vi "log analysis_gps.vi"() -> ()   [LabVIEW 2018] (continued)
normal 2 28.000000 0 0\trobot status\t244.692862\t98.039644\t8.450300\t-0.803805\t-0.502559\t154.815387\t0.298000\t0.012000\n\t\n15:36:08.1\tlog_raw\tgps_raw\t#INSPVAXA,USB3,0,46.5,FINESTEERING,2107,282986.150,02008000,471d,15824;INS_ALIGNMENT_COMPLETE,INS_RTKFIXED,37.37101422818,126.72359615090,8.4473,22.3000,0.1631,-0.2437,-0.0170,-1.039180574,-0.597901795,295.266800009,0.4472,0.2951,0.5600,0.1141,0.0926,0.0776,0.0978,0.1028,4.9255,0f000001,0*b918d4c4\n\tsystem status\tnormal 2 28.000000 0 0\trobot status\t244.568915\t98.110325\t8.447300\t-1.039181\t-0.597902\t154.733200\t0.361000\t-0.105000\n\t\n15:36:08.6\tlog_raw\tgps_raw\t\tsystem status\tnormal 2 27.900000 0 0\trobot status\t244.444418\t98.179771\t8.446900\t-1.452290\t-0.735471\t154.720591\t0.349000\t-0.074000\n\t\n15:36:09.1\tlog_raw\tgps_raw\t\tsystem status\tnormal 2 27.900000 0 0\trobot status\t244.323302\t98.251356\t8.447400\t-1.387904\t-0.757629\t154.772005\t0.295000\t0.004000\n\t\n15:36:09.6\tlog_raw\tgps_raw\t\tsystem status\tnormal 2 27.900000 0 0\trobot status\t244.200377\t98.324148\t8.445900\t-1.199779\t-0.776977\t154.794421\t0.351000\t-0.085000\n\t\n15:36:10.1\tlog_raw\tgps_raw\t#INSPVAXA,USB3,0,51.5,FINESTEERING,2107,282988.150,02000000,471d,15824;INS_ALIGNMENT_COMPLETE,INS_RTKFIXED,37.37101680407,126.72359058877,8.4432,22.3000,0.1712,-0.2477,-0.0072,-1.132987341,-0.795555306,295.241601401,0.4472,0.2951,0.5599,0.1141,0.0926,0.0776,0.0978,0.1028,4.9272,0f000001,0*1b3b971d\n\tsystem status\tnormal 2 28.000000 0 0\trobot status\t244.076230\t98.396223\t8.443200\t-1.132987\t-0.795555\t154.758399\t0.259000\t0.061000\n\t\n15:36:10.6\tlog_raw\tgps_raw\t#INSPVAXA,USB3,0,51.5,FINESTEERING,2107,282988.650,02000000,471d,15824;INS_ALIGNMENT_COMPLETE,INS_RTKFIXED,37.37101744623,126.72358920504,8.4402,22.3000,0.1681,-0.2455,-0.0077,-0.918184944,-0.964879494,295.259837239,0.4472,0.2951,0.5599,0.1141,0.0926,0.0776,0.0978,0.1028,4.9272,0f000001,0*72c9ff23\n\tsystem status\tnormal 2 27.900000 0 0\trobot status\t243.953662\t98.467497\t8.440200\t-0.918185\t-0.964879\t154.740163\t0.282000\t0.015000\n\t\n15:36:11.1\tlog_raw\tgps_raw\t#INSPVAXA,USB3,0,52.0,FINESTEERING,2107,282989.150,02000000,471d,15824;INS_ALIGNMENT_COMPLETE,INS_RTKFIXED,37.37101810010,126.72358780342,8.4378,22.3000,0.1635,-0.2346,-0.0127,-0.821579606,-1.181208357,295.261813725,0.4470,0.2950,0.5598,0.1141,0.0925,0.0776,0.0977,0.1028,4.9279,0f000001,0*084187d8\n\tsystem status\tnormal 2 27.900000 0 0\trobot status\t243.829509\t98.540070\t8.437800\t-0.821580\t-1.181208\t154.738186\t0.346000\t-0.094000\n\t\n15:36:11.6\tlog_raw\tgps_raw\t#INSPVAXA,USB3,0,52.0,FINESTEERING,2107,282989.650,02000000,471d,15824;INS_ALIGNMENT_COMPLETE,INS_RTKFIXED,37.37101876823,126.72358639475,8.4359,22.3000,0.1596,-0.2371,-0.0062,-0.715677130,-1.181942284,295.239523711,0.4470,0.2950,0.5598,0.1141,0.0925,0.0776,0.0977,0.1028,4.9279,0f000001,0*db6d0e7d\n\tsystem status\tnormal 2 28.000000 0 0\trobot status\t243.704731\t98.614226\t8.435900\t-0.715677\t-1.181942\t154.760476\t0.253000\t0.047000\n\t\n15:36:12.1\tlog_raw\tgps_raw\t#INSPVAXA,USB3,0,50.0,FINESTEERING,2107,282990.150,02000000,471d,15824;INS_ALIGNMENT_COMPLETE,INS_RTKFIXED,37.37101943584,126.72358497714,8.4335,22.3000,0.1613,-0.2440,-0.0113,-0.746627018,-1.102743180,295.224075586,0.4466,0.2950,0.5597,0.1141,0.0925,0.0776,0.0977,0.1028,4.9289,0f000001,0*6b0a1647\n\tsystem status\tnormal 2 28.000000 0 0\trobot status\t243.579161\t98.688324\t8.433500\t-0.746627\t-1.102743\t154.775924\t0.282000\t0.033000\n\t\n15:36:12.6\tlog_raw\tgps_raw\t#INSPVAXA,USB3,0,50.0,FINESTEERING,2107,282990.650,02000000,471d,15824;INS_ALIGNMENT_COMPLETE,INS_RTKFIXED,37.37102009853,126.72358357998,8.4311,22.3000,0.1630,-0.2513,-0.0092,-0.640841059,-0.917447835,295.078324917,0.4466,0.2950,0.5597,0.1141,0.0925,0.0776,0.0977,0.1028,4.9289,0f000001,0*b9d8443c\n\tsystem status\tnormal 2 28.000000 0 0\trobot status\t243.455403\t98.761876\t8.431100\t-0.640841\t-0.917448\t154.921675\t0.378000\t-0.109000\n\t\n15:36:13.1\tlog_raw\tgps_raw\t#INSPVAXA,USB3,0,51.0,FINESTEERING,2107,282991.150,02000000,471d,15824;INS_ALIGNMENT_COMPLETE,INS_RTKFIXED,37.37102077697,126.72358217095,8.4272,22.3000,0.1498,-0.2404,-0.0111,-0.329986353,-0.737306515,294.974204977,0.4460,0.2950,0.5595,0.1141,0.0925,0.0776,0.0977,0.1028,4.9303,0f000001,0*44f52417\n\tsystem status\tnormal 2 27.900000 0 0\trobot status\t243.330594\t98.837176\t8.427200\t-0.329986\t-0.737307\t155.025795\t0.275000\t0.036000\n\t\n15:36:13.6\tlog_raw\tgps_raw\t\tsystem status\tnormal 2 27.900000 0 0\trobot status\t243.204049\t98.910416\t8.424600\t-0.403055\t-0.840461\t155.109599\t0.256000\t0.075000\n\t\n15:36:14.1\tlog_raw\tgps_raw\t#INSPVAXA,USB3,0,52.0,FINESTEERING,2107,282992.150,02000000,471d,15824;INS_ALIGNMENT_COMPLETE,INS_RTKFIXED,37.37102208780,126.72357933244,8.4219,22.3000,0.1505,-0.2512,-0.0006,-0.471923349,-0.884947239,294.718584068,0.4460,0.2949,0.5594,0.1141,0.0926,0.0776,0.0977,0.1028,4.9317,0f000001,0*525866c6\n\tsystem status\tnormal 2 27.900000 0 0\trobot status\t243.079163\t98.982665\t8.421900\t-0.471923\t-0.884947\t155.281416\t0.245000\t0.082000\n\t\n15:36:14.6\tlog_raw\tgps_raw\t\tsystem status\tnormal 2 27.900000 0 0\trobot status\t242.954926\t99.054298\t8.420600\t-0.447132\t-0.873245\t155.408066\t0.286000\t0.033000\n\t\n15:36:15.1\tlog_raw\tgps_raw\t\tsystem status\tnormal 2 27.900000 0 0\trobot status\t242.830833\t99.126924\t8.419200\t-0.327815\t-0.760203\t155.517928\t0.356000\t-0.079000\n\t\n15:36:15.6\tlog_raw\tgps_raw\t\tsystem status\tnormal 2 27.900000 0 0\trobot status\t242.705129\t99.198573\t8.417700\t-0.367400\t-0.721993\t155.690211\t0.279000\t0.039000\n\t\n15:36:16.1\tlog_raw\tgps_raw\t\tsystem status\tnormal 2 27.900000 0 0\trobot status\t242.579117\t99.269179\t8.416000\t-0.582357\t-0.735126\t155.797376\t0.243000\t0.086000\n\t\n15:36:16.6\tlog_raw\tgps_raw\t\tsystem status\tnormal 2 27.900000 0 0\trobot status\t242.453519\t99.339670\t8.415000\t-0.617090\t-0.662184\t155.942723\t0.354000\t-0.074000\n\t\n15:36:17.1\tlog_raw\tgps_raw\t\tsystem status\tnormal 2 27.900000 0 0\trobot status\t242.325366\t99.411603\t8.413900\t-0.531047\t-0.781812\t156.112555\t0.222000\t0.108000\n\t\n15:36:17.6\tlog_raw\tgps_raw\t\tsystem status\tnormal 2 27.900000 0 0\trobot status\t242.197882\t99.480396\t8.412000\t-0.574216\t-0.924224\t156.274601\t0.281000\t0.029000\n\t\n15:36:18.1\tlog_raw\tgps_raw\t\tsystem status\tnormal 2 27.900000 0 0\trobot status\t242.070413\t99.549648\t8.409200\t-0.560898\t-1.025999\t156.424077\t0.327000\t-0.033000\n\t\n15:36:18.6\tlog_raw\tgps_raw\t\tsystem status\tnormal 2 27.900000 0 0\trobot status\t241.941493\t99.617825\t8.405800\t-0.542524\t-1.180480\t156.491955\t0.254000\t0.064000\n\t\n15:36:19.1\tlog_raw\tgps_raw\t\tsystem status\tnormal 2 27.900000 0 0\trobot status\t241.811834\t99.686587\t8.402800\t-0.566001\t-1.561653\t156.587783\t0.260000\t0.056000\n\t\n15:36:19.6\tlog_raw\tgps_raw\t\tsystem status\tnormal 2 27.900000 0 0\trobot status\t241.684911\t99.755728\t8.400600\t-0.615139\t-1.607167\t156.703459\t0.290000\t0.026000\n\t\n15:36:20.1\tlog_raw\tgps_raw\t\tsystem status\tnormal 2 27.900000 0 0\trobot status\t241.559726\t99.825209\t8.399300\t-0.552219\t-1.574627\t156.768165\t0.262000\t0.066000\n\t\n15:36:20.6\tlog_raw\tgps_raw\t\tsystem status\tnormal 2 27.900000 0 0\trobot status\t241.433525\t99.894376\t8.397900\t-0.537757\t-1.498689\t156.817308\t0.339000\t-0.045000\n\t\n15:36:21.1\tlog_raw\tgps_raw\t\tsystem status\tnormal 2 27.900000 0 0\trobot status\t241.309976\t99.962850\t8.395200\t-0.464581\t-1.180262\t156.857945\t0.334000\t-0.044000\n\t\n15:36:21.6\tlog_raw\tgps_raw\t\tsystem status\tnormal 2 27.900000 0 0\trobot status\t241.187325\t100.030799\t8.392900\t-0.376983\t-1.123165\t156.922194\t0.223000\t0.121000\n\t\n15:36:22.1\tlog_raw\tgps_raw\t#INSPVAXA,USB3,0,42.5,FINESTEERING,2107,283000.150,02008000,471d,15824;INS_ALIGNMENT_COMPLETE,INS_RTKFIXED,37.37103215127,126.72355655993,8.3901,22.3000,0.1524,-0.2449,-0.0003,-0.362652962,-1.080137119,293.057786334,0.4445,0.2951,0.5592,0.1140,0.0926,0.0776,0.0977,0.1028,4.9425,0f000001,0*4235a1eb\n\tsystem status\tnormal 2 28.000000 0 0\trobot status\t241.062012\t100.099614\t8.390100\t-0.362653\t-1.080137\t156.942214\t0.357000\t-0.096000\n\t\n15:36:22.6\tlog_raw\tgps_raw\t\tsystem status\tnormal 2 28.000000 0 0\trobot status\t240.934705\t100.169062\t8.388500\t-0.314213\t-1.316526\t156.995133\t0.237000\t0.069000\n\t\n15:36:23.1\tlog_raw\tgps_raw\t\tsystem status\tnormal 2 28.000000 0 0\trobot status\t240.809010\t100.237494\t8.386700\t-0.267509\t-1.341608\t157.070363\t0.307000\t0.007000\n\t\n15:36:23.6\tlog_raw\tgps_raw\t\tsystem status\tnormal 2 27.900000 0 0\trobot status\t240.686600\t100.302527\t8.386000\t-0.209028\t-1.240600\t157.178946\t0.374000\t-0.108000\n\t\n15:36:24.1\tlog_raw\tgps_raw\t\tsystem status\tnormal 2 27.900000 0 0\trobot status\t240.561796\t100.368931\t8.383800\t-0.114387\t-1.159675\t157.312989\t0.298000\t-0.019000\n\t\n15:36:24.6\tlog_raw\tgps_raw\t\tsystem status\tnormal 2 27.900000 0 0\trobot status\t240.435903\t100.435393\t8.381400\t-0.172130\t-1.043551\t157.446511\t0.220000\t0.117000\n\t\n15:36:25.1\tlog_raw\tgps_raw\t\tsystem status\tnormal 2 27.900000 0 0\trobot status\t240.309740\t100.501734\t8.378200\t-0.129443\t-1.017241\t157.594683\t0.348000\t-0.088000\n\t\n15:36:25.6\tlog_raw\tgps_raw\t#INSPVAXA,USB3,0,49.0,FINESTEERING,2107,283003.650,02008000,471d,15824;INS_ALIGNMENT_COMPLETE,INS_RTKFIXED,37.37103636428,126.72354662832,8.3755,22.3000,0.1350,-0.2615,-0.0053,-0.069883534,-0.948015743,292.302597203,0.4446,0.2951,0.5590,0.1140,0.0925,0.0776,0.0978,0.1028,4.9465,0f000001,0*59130eb8\n\tsystem status\tnormal 2 27.900000 0 0\trobot status\t240.182286\t100.567218\t8.375500\t-0.069884\t-0.948016\t157.697403\t0.347000\t-0.082000\n\t\n15:36:26.1\tlog_raw\tgps_raw\t\tsystem status\tnormal 2 27.900000 0 0\trobot status\t240.051657\t100.633146\t8.372800\t-0.173374\t-1.126467\t157.829281\t0.280000\t0.015000\n\t\n15:36:26.7\tlog_raw\tgps_raw\t\tsystem status\tnormal 2 27.900000 0 0\trobot status\t239.922071\t100.698890\t8.370700\t-0.264071\t-1.188422\t158.025138\t0.283000\t0.034000\n\t\n15:36:27.2\tlog_raw\tgps_raw\t\tsystem status\tnormal 2 27.900000 0 0\trobot status\t239.792839\t100.765236\t8.368100\t-0.305352\t-1.271586\t158.094882\t0.339000\t-0.062000\n\t\n15:36:27.6\tlog_raw\tgps_raw\t\tsystem status\tnormal 2 27.900000 0 0\trobot status\t239.663623\t100.830918\t8.366100\t-0.343211\t-1.324235\t158.195980\t0.450000\t-0.229000\n\t\n15:36:28.2\tlog_raw\tgps_raw\t\tsystem status\tnormal 2 27.900000 0 0\trobot status\t239.534352\t100.896705\t8.364200\t-0.314060\t-1.319994\t158.324136\t0.257000\t0.072000\n\t\n15:36:28.7\tlog_raw\tgps_raw\t\tsystem status\tnormal 2 27.900000 0 0\trobot status\t239.406547\t100.960925\t8.362500\t-0.258928\t-1.174312\t158.404351\t0.381000\t-0.103000\n\t\n15:36:29.1\tlog_raw\tgps_raw\t\tsystem status\tnormal 2 27.900000 0 0\trobot status\t239.277688\t101.025267\t8.359900\t-0.293969\t-1.010654\t158.496365\t0.346000\t-0.059000\n\t\n15:36:29.6\tlog_raw\tgps_raw\t\tsystem status\tnormal 2 27.900000 0 0\trobot status\t239.148045\t101.088847\t8.357100\t-0.431958\t-0.959264\t158.582891\t0.287000\t0.019000\n\t\n15:36:30.2\tlog_raw\tgps_raw\t\tsystem status\tnormal 2 27.900000 0 0\trobot status\t239.019804\t101.152841\t8.355200\t-0.465469\t-0.805617\t158.766817\t0.372000\t-0.098000\n\t\n15:36:30.6\tlog_raw\tgps_raw\t\tsystem status\tnormal 2 27.900000 0 0\trobot status\t238.892777\t101.217417\t8.354000\t-0.368318\t-0.774393\t158.922796\t0.341000\t-0.059000\n\t\n15:36:31.1\tlog_raw\tgps_raw\t\tsystem status\tnormal 2 27.900000 0 0\trobot status\t238.763580\t101.282027\t8.352100\t-0.373752\t-0.757788\t159.085038\t0.222000\t0.122000\n\t\n15:36:31.7\tlog_raw\tgps_raw\t\tsystem status\tnormal 2 27.900000 0 0\trobot status\t238.634583\t101.344929\t8.350300\t-0.519696\t-0.590256\t159.213603\t0.342000\t-0.067000\n\t\n15:36:32.2\tlog_raw\tgps_raw\t\tsystem status\tnormal 2 27.900000 0 0\trobot status\t238.504480\t101.407745\t8.349200\t-0.610956\t-0.693965\t159.324003\t0.224000\t0.115000\n\t\n15:36:32.6\tlog_raw\tgps_raw\t\tsystem status\tnormal 2 27.900000 0 0\trobot status\t238.374891\t101.469502\t8.348000\t-0.622591\t-0.731069\t159.487231\t0.209000\t0.143000\n\t\n15:36:33.1\tlog_raw\tgps_raw\t\tsystem status\tnormal 2 27.900000 0 0\trobot status\t238.244641\t101.530850\t8.346700\t-0.723407\t-0.771971\t159.667053\t0.366000\t-0.093000\n\t\n15:36:33.7\tlog_raw\tgps_raw\t\tsystem status\tnormal 2 27.900000 0 0\trobot status\t238.115486\t101.591392\t8.347000\t-0.788066\t-0.747634\t159.858332\t0.281000\t0.037000\n\t\n15:36:34.1\tlog_raw\tgps_raw\t\tsystem status\tnormal 2 27.900000 0 0\trobot status\t237.986285\t101.650207\t8.346900\t-0.994357\t-0.650902\t159.990881\t0.215000\t0.129000\n\t\n15:36:34.6\tlog_raw\tgps_raw\t\tsystem status\tnormal 2 27.900000 0 0\trobot status\t237.858246\t101.709402\t8.345300\t-1.038620\t-0.473997\t160.049241\t0.248000\t0.082000\n\t\n15:36:35.2\tlog_raw\tgps_raw\t\tsystem status\tnormal 2 27.900000 0 0\trobot status\t237.728450\t101.768656\t8.343900\t-1.062118\t-0.508142\t160.161998\t0.278000\t0.032000\n\t\n15:36:35.7\tlog_raw\tgps_raw\t\tsystem status\tnormal 2 28.000000 0 0\trobot status\t237.599188\t101.827012\t8.344700\t-1.031691\t-0.580801\t160.225175\t0.210000\t0.139000\n\t\n15:36:36.2\tlog_raw\tgps_raw\t\tsystem status\tnormal 2 27.900000 0 0\trobot status\t237.468929\t101.885123\t8.345300\t-1.104431\t-0.651052\t160.247354\t0.258000\t0.060000\n\t\n15:36:36.7\tlog_raw\tgps_raw\t\tsystem status\tnormal 2 27.900000 0 0\trobot status\t237.338972\t101.943812\t8.346400\t-1.199680\t-0.770269\t160.324632\t0.349000\t-0.074000\n\t\n15:36:37.2\tlog_raw\tgps_raw\t\tsystem status\tnormal 2 28.000000 0 0\trobot status\t237.221978\t101.998401\t8.345800\t-1.189265\t-0.855125\t160.431147\t0.218000\t-0.049000\n\t\n15:36:37.7\tlog_raw\tgps_raw\t\tsystem status\tnormal 2 28.000000 0 0\trobot status\t237.096804\t102.054564\t8.343700\t-1.253495\t-1.073832\t160.664044\t0.100000\t0.026000\n\t\n15:36:38.2\tlog_raw\tgps_raw\t\tsystem status\tnormal 2 28.000000 0 0\trobot status\t237.101789\t102.065438\t8.342300\t-1.271823\t-0.943171\t160.404484\t-0.006000\t0.009000\n\t\n15:36:38.7\tlog_raw\tgps_raw\t\tsystem status\tnormal 2 28.000000 0 0\trobot status\t237.105323\t102.074573\t8.340600\t-1.267963\t-0.940917\t160.442539\t0.000000\t0.000000\n\t\n15:36:39.2\tlog_raw\tgps_raw\t\tsystem status\tnormal 2 27.800000 0 0\trobot status\t237.064766\t102.097094\t8.339200\t-1.261431\t-0.757005\t160.638796\t0.323000\t0.006000\n\t\n15:36:39.7\tlog_raw\tgps_raw\t\tsystem status\tnormal 2 28.000000 0 0\trobot status\t236.897456\t102.162973\t8.336000\t-1.010954\t-1.103124\t160.428503\t0.335000\t-0.062000\n\t\n15:36:40.2\tlog_raw\tgps_raw\t\tsystem status\tnormal 2 27.900000 0 0\trobot status\t236.781475\t102.209572\t8.333900\t-1.044765\t-1.121813\t160.397624\t0.322000\t0.027000\n\t\n15:36:40.7\tlog_raw\tgps_raw\t\tsystem status\tnormal 2 27.900000 0 0\trobot status\t236.645564\t102.268025\t8.331200\t-1.001377\t-1.191370\t160.289169\t0.251000\t0.040000\n\t\n15:36:41.2\tlog_raw\tgps_raw\t\tsystem status\tnormal 2 28.000000 0 0\trobot status\t236.507116\t102.326660\t8.328000\t-1.123546\t-1.162038\t160.257441\t0.357000\t-0.074000\n\t\n15:36:41.7\tlog_raw\tgps_raw\t\tsystem status\tnormal 2 28.000000 0 0\trobot status\t236.378362\t102.382583\t8.324500\t-1.141056\t-1.061916\t160.353991\t0.382000\t-0.094000\n\t\n15:36:42.2\tlog_raw\tgps_raw\t\tsystem status\tnormal 2 27.900000 0 0\trobot status\t236.248466\t102.439596\t8.320600\t-1.042246\t-1.070351\t160.529344\t0.372000\t-0.090000\n\t\n15:36:42.7\tlog_raw\tgps_raw\t\tsystem status\tnormal 2 27.900000 0 0\trobot status\t236.114925\t102.499303\t8.316500\t-0.817092\t-1.153049\t160.650639\t0.325000\t-0.032000\n\t\n15:36:43.2\tlog_raw\tgps_raw\t\tsystem status\tnormal 2 27.900000 0 0\trobot status\t235.982387\t102.558482\t8.313000\t-0.647908\t-1.305675\t160.819142\t0.224000\t0.112000\n\t\n15:36:43.7\tlog_raw\tgps_raw\t#INSPVAXA,USB3,0,51.0,FINESTEERING,2107,283021.700,02000000,471d,15824;INS_ALIGNMENT_COMPLETE,INS_RTKFIXED,37.37105488806,126.72349758761,8.3107,22.3000,0.1124,-0.2877,-0.0191,-0.603845157,-1.428014368,288.935954178,0.4473,0.2957,0.5615,0.1144,0.0929,0.0777,0.0976,0.1028,4.9397,0f000001,0*95301355\n\tsystem status\tnormal 2 27.900000 0 0\trobot status\t235.838340\t102.623197\t8.310700\t-0.603845\t-1.428014\t161.064046\t0.313000\t-0.015000\n\t\n15:36:44.2\tlog_raw\tgps_raw\t\tsystem status\tnormal 2 27.900000 0 0\trobot status\t235.718631\t102.677526\t8.308000\t-0.474030\t-1.589082\t161.226491\t0.352000\t-0.070000\n\t\n15:36:44.7\tlog_raw\tgps_raw\t\tsystem status\tnormal 2 27.900000 0 0\trobot status\t235.587048\t102.737395\t8.306300\t-0.316912\t-1.512041\t161.525838\t0.260000\t0.059000\n\t\n15:36:45.2\tlog_raw\tgps_raw\t\tsystem status\tnormal 2 27.900000 0 0\trobot status\t235.459193\t102.794680\t8.305200\t-0.318622\t-1.185691\t161.878516\t0.317000\t-0.003000\n\t\n15:36:45.7\tlog_raw\tgps_raw\t\tsystem status\tnormal 2 27.900000 0 0\trobot status\t235.330595\t102.852240\t8.303600\t-0.250164\t-0.969800\t162.178967\t0.285000\t0.042000\n\t\n15:36:46.2\tlog_raw\tgps_raw\t\tsystem status\tnormal 2 27.900000 0 0\trobot status\t235.199534\t102.911305\t8.300800\t-0.038583\t-0.774737\t162.476073\t0.198000\t0.152000\n\t\n15:36:46.7\tlog_raw\tgps_raw\t\tsystem status\tnormal 2 27.900000 0 0\trobot status\t235.070719\t102.969017\t8.299000\t0.203261\t-0.566713\t162.738097\t0.343000\t-0.058000\n\t\n15:36:47.2\tlog_raw\tgps_raw\t\tsystem status\tnormal 2 27.900000 0 0\trobot status\t234.942040\t103.025794\t8.298600\t0.179760\t-0.475961\t162.985067\t0.300000\t-0.016000\n\t\n15:36:47.7\tlog_raw\tgps_raw\t\tsystem status\tnormal 2 27.900000 0 0\trobot status\t234.810405\t103.083318\t8.299100\t0.078958\t-0.377098\t163.210942\t0.335000\t-0.033000\n\t\n15:36:48.2\tlog_raw\tgps_raw\t#INSPVAXA,USB3,0,49.5,FINESTEERING,2107,283026.200,02000000,471d,15824;INS_ALIGNMENT_COMPLETE,INS_RTKFIXED,37.37105960737,126.72348434447,8.2980,22.3000,0.1329,-0.2636,-0.0189,0.063004840,-0.340709655,286.479818282,0.4478,0.2967,0.5618,0.1144,0.0930,0.0777,0.0976,0.1028,4.9376,0f000001,0*1276055f\n\tsystem status\tnormal 2 27.900000 0 0\trobot status\t234.665284\t103.147000\t8.298000\t0.063005\t-0.340710\t163.520182\t0.225000\t0.120000\n\t\n15:36:48.7\tlog_raw\tgps_raw\t#INSPVAXA,USB3,0,49.5,FINESTEERING,2107,283026.700,02000000,471d,15824;INS_ALIGNMENT_COMPLETE,INS_RTKFIXED,37.37106011573,126.72348287105,8.2978,22.3000,0.1361,-0.2641,-0.0054,0.117267102,-0.429574615,286.158968157,0.4478,0.2967,0.5618,0.1144,0.0930,0.0777,0.0976,0.1028,4.9376,0f000001,0*5e7b6e4c\n\tsystem status\tnormal 2 27.800000 0 0\trobot status\t234.534771\t103.203424\t8.297800\t0.117267\t-0.429575\t163.841032\t0.274000\t0.055000\n\t\n15:36:49.2\tlog_raw\tgps_raw\t\tsystem status\tnormal 2 27.900000 0 0\trobot status\t234.417219\t103.253409\t8.298000\t0.090142\t-0.537319\t164.032490\t0.287000\t0.024000\n\t\n15:36:49.7\tlog_raw\tgps_raw\t\tsystem status\tnormal 2 27.900000 0 0\trobot status\t234.284444\t103.307798\t8.297800\t0.078625\t-0.685486\t164.310887\t0.258000\t0.068000\n\t\n15:36:50.2\tlog_raw\tgps_raw\t\tsystem status\tnormal 2 27.900000 0 0\trobot status\t234.150560\t103.364212\t8.295600\t0.061664\t-0.774003\t164.542735\t0.261000\t0.058000\n\t\n15:36:50.7\tlog_raw\tgps_raw\t#INSPVAXA,USB3,0,51.0,FINESTEERING,2107,283028.700,02000000,471d,15824;INS_ALIGNMENT_COMPLETE,INS_RTKFIXED,37.37106216690,126.72347687588,8.2864,22.3000,0.1309,-0.2689,-0.0192,0.186843092,-0.733613346,285.184747118,0.4481,0.2969,0.5618,0.1144,0.0930,0.0777,0.0976,0.1028,4.9364,0f000001,0*7469a4e3\n\tsystem status\tnormal 2 27.900000 0 0\trobot status\t234.003729\t103.431087\t8.286400\t0.186843\t-0.733613\t164.815253\t0.209000\t0.128000\n\t\n15:36:51.2\tlog_raw\tgps_raw\t\tsystem status\tnormal 2 27.900000 0 0\trobot status\t233.882277\t103.482746\t8.281200\t0.229624\t-0.607695\t165.093813\t0.235000\t0.090000\n\t\n15:36:51.7\tlog_raw\tgps_raw\t\tsystem status\tnormal 2 27.900000 0 0\trobot status\t233.749301\t103.532863\t8.281500\t0.339876\t-0.636036\t165.368673\t0.251000\t0.085000\n\t\n15:36:52.2\tlog_raw\tgps_raw\t\tsystem status\tnormal 2 27.800000 0 0\trobot status\t233.616889\t103.581753\t8.280300\t0.438301\t-0.662131\t165.694482\t0.289000\t0.011000\n\t\n15:36:52.7\tlog_raw\tgps_raw\t\tsystem status\tnormal 2 27.900000 0 0\trobot status\t233.481222\t103.627529\t8.277000\t0.356298\t-0.796827\t166.034479\t0.281000\t0.036000\n\t\n15:36:53.2\tlog_raw\tgps_raw\t\tsystem status\tnormal 2 27.900000 0 0\trobot status\t233.345075\t103.673571\t8.273700\t0.373415\t-0.855267\t166.315058\t0.271000\t0.051000\n\t\n15:36:53.7\tlog_raw\tgps_raw\t#INSPVAXA,USB3,0,50.5,FINESTEERING,2107,283031.700,02000000,471d,15824;INS_ALIGNMENT_COMPLETE,INS_RTKFIXED,37.37106478537,126.72346780785,8.2718,22.3000,0.1039,-0.2615,-0.0058,0.432632982,-0.697195774,283.403693231,0.4679,0.3078,0.5901,0.1164,0.0946,0.0783,0.0984,0.1034,4.9333,0f000001,0*22ba6c5b\n\tsystem status\tnormal 2 27.900000 0 0\trobot status\t233.200498\t103.721720\t8.271800\t0.432633\t-0.697196\t166.596307\t0.244000\t0.093000\n\t\n15:36:54.2\tlog_raw\tgps_raw\t\tsystem status\tnormal 2 27.900000 0 0\trobot status\t233.081426\t103.761828\t8.269700\t0.599537\t-0.465596\t166.852966\t0.487000\t-0.272000\n\t\n15:36:54.7\tlog_raw\tgps_raw\t#INSPVAXA,USB3,0,52.5,FINESTEERING,2107,283032.700,02000000,471d,15824;INS_ALIGNMENT_COMPLETE,INS_RTKFIXED,37.37106557652,126.72346477114,8.2666,22.3000,0.1036,-0.2653,-0.0227,0.510573664,-0.506867752,282.989814532,0.4595,0.3023,0.5832,0.1161,0.0945,0.0778,0.0983,0.1032,4.9326,0f000001,0*f19d58ff\n\tsystem status\tnormal 2 27.900000 0 0\trobot status\t232.931511\t103.809533\t8.266600\t0.510574\t-0.506868\t167.010185\t0.278000\t0.025000\n\t\n15:36:55.2\tlog_raw\tgps_raw\t#INSPVAXA,USB3,0,49.5,FINESTEERING,2107,283033.200,02000000,471d,15824;INS_ALIGNMENT_COMPLETE,INS_RTKFIXED,37.37106596612,126.72346326783,8.2630,22.3000,0.1080,-0.2670,-0.0291,0.451082003,-0.356947315,282.881862782,0.4543,0.2994,0.5774,0.1160,0.0946,0.0775,0.0983,0.1032,4.9319,0f000001,0*26a02b0e\n\tsystem status\tnormal 2 27.900000 0 0\trobot status\t232.798350\t103.852776\t8.263000\t0.451082\t-0.356947\t167.118137\t0.355000\t-0.076000\n\t\n15:36:55.7\tlog_raw\tgps_raw\t#INSPVAXA,USB3,0,49.5,FINESTEERING,2107,283033.700,02000000,471d,15824;INS_ALIGNMENT_COMPLETE,INS_RTKFIXED,37.37106635735,126.72346178545,8.2608,22.3000,0.1136,-0.2627,-0.0166,0.359711972,-0.310104269,282.738479610,0.4543,0.2994,0.5774,0.1160,0.0946,0.0775,0.0983,0.1032,4.9319,0f000001,0*88f043a8\n\tsystem status\tnormal 2 27.900000 0 0\trobot status\t232.667043\t103.896200\t8.260800\t0.359712\t-0.310104\t167.261520\t0.243000\t0.065000\n\t\n15:36:56.2\tlog_raw\tgps_raw\t#INSPVAXA,USB3,0,50.0,FINESTEERING,2107,283034.200,02000000,471d,15824;INS_ALIGNMENT_COMPLETE,INS_RTKFIXED,37.37106676961,126.72346024394,8.2592,22.3000,0.1183,-0.2649,-0.0209,0.421889182,-0.508488076,282.654292643,0.4522,0.2981,0.5733,0.1161,0.0947,0.0774,0.0982,0.1031,4.9317,0f000001,0*726c30e6\n\tsystem status\tnormal 2 27.900000 0 0\trobot status\t232.530499\t103.941958\t8.259200\t0.421889\t-0.508488\t167.345707\t0.340000\t-0.069000\n\t\n15:36:56.7\tlog_raw\tgps_raw\t#INSPVAXA,USB3,0,50.0,FINESTEERING,2107,283034.700,02000000,471d,15824;INS_ALIGNMENT_COMPLETE,INS_RTKFIXED,37.37106718417,126.72345866239,8.2575,22.3000,0.1236,-0.2716,-0.0253,0.328679874,-0.657327214,282.636912326,0.4522,0.2981,0.5733,0.1161,0.0947,0.0774,0.0982,0.1031,4.9317,0f000001,0*dafccd04\n\tsystem status\tnormal 2 27.900000 0 0\trobot status\t232.390408\t103.987972\t8.257500\t0.328680\t-0.657327\t167.363088\t0.381000\t-0.117000\n\t\n15:36:57.2\tlog_raw\tgps_raw\t\tsystem status\tnormal 2 27.900000 0 0\trobot status\t232.270676\t104.028905\t8.256900\t0.332540\t-0.618431\t167.360994\t0.282000\t0.017000\n\t\n15:36:57.7\tlog_raw\tgps_raw\t#INSPVAXA,USB3,0,51.5,FINESTEERING,2107,283035.700,02000000,471d,15824;INS_ALIGNMENT_COMPLETE,INS_RTKFIXED,37.37106801887,126.72345563034,8.2572,22.3000,0.1130,-0.2756,-0.0204,0.415680763,-0.663146302,282.634386607,0.4503,0.2974,0.5697,0.1160,0.0945,0.0774,0.0981,0.1030,4.9320,0f000001,0*eab13697\n\tsystem status\tnormal 2 27.900000 0 0\trobot status\t232.121834\t104.080618\t8.257200\t0.415681\t-0.663146\t167.365613\t0.293000\t0.013000\n\t\n15:36:58.2\tlog_raw\tgps_raw\t#INSPVAXA,USB3,0,40.5,FINESTEERING,2107,283036.200,02000000,471d,15824;INS_ALIGNMENT_COMPLETE,INS_RTKFIXED,37.37106843656,126.72345404474,8.2574,22.3000,0.1206,-0.2843,-0.0254,0.323424961,-0.903914329,282.663197732,0.4498,0.2973,0.5674,0.1161,0.0943,0.0774,0.0979,0.1030,4.9328,0f000001,0*9733e7d0\n\tsystem status\tnormal 2 27.900000 0 0\trobot status\t231.981384\t104.126979\t8.257400\t0.323425\t-0.903914\t167.336802\t0.365000\t-0.092000\n\t\n15:36:58.7\tlog_raw\tgps_raw\t#INSPVAXA,USB3,0,40.5,FINESTEERING,2107,283036.700,02000000,471d,15824;INS_ALIGNMENT_COMPLETE,INS_RTKFIXED,37.37106883526,126.72345250109,8.2575,22.3000,0.1230,-0.2819,-0.0264,0.242869357,-1.036611365,282.652291179,0.4498,0.2973,0.5674,0.1161,0.0943,0.0774,0.0979,0.1030,4.9328,0f000001,0*470d739a\n\tsystem status\tnormal 2 27.900000 0 0\trobot status\t231.844650\t104.171233\t8.257500\t0.242869\t-1.036611\t167.347709\t0.361000\t-0.087000\n\t\n15:36:59.2\tlog_raw\tgps_raw\t#INSPVAXA,USB3,0,48.5,FINESTEERING,2107,283037.200,02000000,471d,15824;INS_ALIGNMENT_COMPLETE,INS_RTKFIXED,37.37106923446,126.72345098005,8.2563,22.3000,0.1194,-0.2683,-0.0234,0.058649364,-1.081028775,282.621575869,0.4494,0.2971,0.5657,0.1160,0.0940,0.0775,0.0978,0.1029,4.9342,0f000001,0*f5724e44\n\tsystem status\tnormal 2 27.900000 0 0\trobot status\t231.709919\t104.215542\t8.256300\t0.058649\t-1.081029\t167.378424\t0.272000\t0.029000\n\t\n15:36:59.7\tlog_raw\tgps_raw\t#INSPVAXA,USB3,0,48.5,FINESTEERING,2107,283037.700,02000000,471d,15824;INS_ALIGNMENT_COMPLETE,INS_RTKFIXED,37.37106966075,126.72344944048,8.2560,22.3000,0.1291,-0.2596,-0.0199,0.104783484,-1.127316645,282.608621596,0.4494,0.2971,0.5657,0.1160,0.0940,0.0775,0.0978,0.1029,4.9342,0f000001,0*8aba2554\n\tsystem status\tnormal 2 27.900000 0 0\trobot status\t231.573546\t104.262857\t8.256000\t0.104783\t-1.127317\t167.391378\t0.366000\t-0.106000\n\t\n15:37:00.2\tlog_raw\tgps_raw\t\tsystem status\tnormal 2 27.900000 0 0\trobot status\t231.449888\t104.305687\t8.255900\t0.128555\t-1.116495\t167.339110\t0.378000\t-0.106000\n\t\n15:37:00.7\tlog_raw\tgps_raw\t\tsystem status\tnormal 2 27.900000 0 0\trobot status\t231.317197\t104.352054\t8.256300\t0.218345\t-1.103930\t167.398981\t0.298000\t0.005000\n\t\n15:37:01.2\tlog_raw\tgps_raw\t#INSPVAXA,USB3,0,50.0,FINESTEERING,2107,283039.200,02000000,471d,15824;INS_ALIGNMENT_COMPLETE,INS_RTKFIXED,37.37107093141,126.72344485682,8.2573,22.3000,0.1183,-0.2711,-0.0111,0.295639650,-1.102682519,282.550490605,0.4487,0.2965,0.5633,0.1155,0.0932,0.0777,0.0976,0.1027,4.9372,0f000001,0*f4702847\n\tsystem status\tnormal 2 27.900000 0 0\trobot status\t231.167533\t104.403892\t8.257300\t0.295640\t-1.102683\t167.449509\t0.327000\t-0.051000\n\t\n15:37:01.7\tlog_raw\tgps_raw\t#INSPVAXA,USB3,0,50.0,FINESTEERING,2107,283039.700,02000000,471d,15824;INS_ALIGNMENT_COMPLETE,INS_RTKFIXED,37.37107133986,126.72344327017,8.2583,22.3000,0.1271,-0.2797,-0.0164,0.252258898,-1.289319637,282.440116082,0.4487,0.2965,0.5633,0.1155,0.0932,0.0777,0.0976,0.1027,4.9372,0f000001,0*06a83079\n\tsystem status\tnormal 2 27.900000 0 0\trobot status\t231.026990\t104.449228\t8.258300\t0.252259\t-1.289320\t167.559884\t0.335000\t-0.061000\n\t\n15:37:02.2\tlog_raw\tgps_raw\t#INSPVAXA,USB3,0,50.0,FINESTEERING,2107,283040.200,02000000,471d,15824;INS_ALIGNMENT_COMPLETE,INS_RTKFIXED,37.37107175331,126.72344170516,8.2593,22.3000,0.1172,-0.2595,-0.0203,0.374259867,-1.387302734,282.178298853,0.4482,0.2962,0.5625,0.1153,0.0929,0.0777,0.0976,0.1026,4.9387,0f000001,0*b656771f\n\tsystem status\tnormal 2 27.900000 0 0\trobot status\t230.888364\t104.495118\t8.259300\t0.374260\t-1.387303\t167.821701\t0.242000\t0.102000\n\t\n15:37:02.7\tlog_raw\tgps_raw\t#INSPVAXA,USB3,0,50.0,FINESTEERING,2107,283040.700,02000000,471d,15824;INS_ALIGNMENT_COMPLETE,INS_RTKFIXED,37.37107213898,126.72344017293,8.2600,22.3000,0.1126,-0.2759,-0.0195,0.475030842,-1.266134141,281.998723158,0.4482,0.2962,0.5625,0.1153,0.0929,0.0777,0.0976,0.1026,4.9387,0f000001,0*1f5b23a7\n\tsystem status\tnormal 2 27.900000 0 0\trobot status\t230.766581\t104.533369\t8.260000\t0.437030\t-1.255302\t167.973588\t0.258000\t0.060000\n\t\n15:37:03.2\tlog_raw\tgps_raw\t#INSPVAXA,USB3,0,45.0,FINESTEERING,2107,283041.200,02000000,471d,15824;INS_ALIGNMENT_COMPLETE,INS_RTKFIXED,37.37107252297,126.72343860548,8.2602,22.3000,0.1112,-0.2748,-0.0176,0.520519283,-1.356863437,281.705665102,0.4477,0.2959,0.5620,0.1149,0.0927,0.0778,0.0976,0.1026,4.9400,0f000001,0*79559378\n\tsystem status\tnormal 2 27.900000 0 0\trobot status\t230.613800\t104.580546\t8.260200\t0.520519\t-1.356863\t168.294335\t0.413000\t-0.162000\n\t\n15:37:03.7\tlog_raw\tgps_raw\t#INSPVAXA,USB3,0,45.0,FINESTEERING,2107,283041.700,02000000,471d,15824;INS_ALIGNMENT_COMPLETE,INS_RTKFIXED,37.37107290097,126.72343701394,8.2600,22.3000,0.1062,-0.2671,-0.0203,0.682698215,-1.388086535,281.490437420,0.4477,0.2959,0.5620,0.1149,0.0927,0.0778,0.0976,0.1026,4.9400,0f000001,0*78dbf0af\n\tsystem status\tnormal 2 27.900000 0 0\trobot status\t230.472824\t104.622502\t8.260000\t0.682698\t-1.388087\t168.509563\t0.250000\t0.078000\n\t\n15:37:04.2\tlog_raw\tgps_raw\t#INSPVAXA,USB3,0,45.5,FINESTEERING,2107,283042.200,02000000,471d,15824;INS_ALIGNMENT_COMPLETE,INS_RTKFIXED,37.37107326636,126.72343547606,8.2588,22.3000,0.1093,-0.2758,-0.0183,0.747095346,-1.168799839,281.251721154,0.4473,0.2957,0.5618,0.1147,0.0926,0.0778,0.0976,0.1026,4.9413,0f000001,0*2a17f75d\n\tsystem status\tnormal 2 27.900000 0 0\trobot status\t230.336601\t104.663058\t8.258800\t0.747095\t-1.168800\t168.748279\t0.344000\t-0.060000\n\t\n15:37:04.7\tlog_raw\tgps_raw\t#INSPVAXA,USB3,0,45.5,FINESTEERING,2107,283042.700,02000000,471d,15824;INS_ALIGNMENT_COMPLETE,INS_RTKFIXED,37.37107361520,126.72343393571,8.2583,22.3000,0.0948,-0.2791,-0.0077,0.665887497,-1.134840592,281.023360507,0.4473,0.2957,0.5618,0.1147,0.0926,0.0778,0.0976,0.1026,4.9413,0f000001,0*de2961a5\n\tsystem status\tnormal 2 27.900000 0 0\trobot status\t230.200159\t104.701778\t8.258300\t0.665887\t-1.134841\t168.976639\t0.290000\t0.012000\n\t\n15:37:05.2\tlog_raw\tgps_raw\t#INSPVAXA,USB3,0,45.5,FINESTEERING,2107,283043.200,02000000,471d,15824;INS_ALIGNMENT_COMPLETE,INS_RTKFIXED,37.37107395395,126.72343236915,8.2577,22.3000,0.0931,-0.2659,-0.0049,0.487857559,-1.159051865,280.826329079,0.4472,0.2955,0.5619,0.1145,0.0925,0.0779,0.0977,0.1026,4.9425,0f000001,0*06efa692\n\tsystem status\tnormal 2 27.900000 0 0\trobot status\t230.061396\t104.739378\t8.257700\t0.487858\t-1.159052\t169.173671\t0.248000\t0.069000\n\t\n15:37:05.7\tlog_raw\tgps_raw\t#INSPVAXA,USB3,0,45.5,FINESTEERING,2107,283043.700,02000000,471d,15824;INS_ALIGNMENT_COMPLETE,INS_RTKFIXED,37.37107428662,126.72343081441,8.2573,22.3000,0.0965,-0.2862,-0.0130,0.491699784,-1.201692637,280.563355107,0.4472,0.2955,0.5619,0.1145,0.0925,0.0779,0.0977,0.1026,4.9425,0f000001,0*ec772638\n\tsystem status\tnormal 2 27.900000 0 0\trobot status\t229.923679\t104.776303\t8.257300\t0.491700\t-1.201693\t169.436645\t0.291000\t0.018000\n\t\n15:37:06.2\tlog_raw\tgps_raw\t#INSPVAXA,USB3,0,49.5,FINESTEERING,2107,283044.200,02000000,471d,15824;INS_ALIGNMENT_COMPLETE,INS_RTKFIXED,37.37107460279,126.72342927244,8.2555,22.3000,0.0952,-0.2841,-0.0084,0.223988399,-1.263049890,280.433215030,0.4470,0.2954,0.5621,0.1143,0.0926,0.0779,0.0977,0.1026,4.9439,0f000001,0*7d3e34bc\n\tsystem status\tnormal 2 27.900000 0 0\trobot status\t229.787094\t104.811397\t8.255500\t0.223988\t-1.263050\t169.566785\t0.249000\t0.067000\n\t\n15:37:06.7\tlog_raw\tgps_raw\t#INSPVAXA,USB3,0,49.5,FINESTEERING,2107,283044.700,02000000,471d,15824;INS_ALIGNMENT_COMPLETE,INS_RTKFIXED,37.37107493652,126.72342768887,8.2530,22.3000,0.0917,-0.2710,-0.0218,0.103359627,-1.313771088,280.424386340,0.4470,0.2954,0.5621,0.1143,0.0926,0.0779,0.0977,0.1026,4.9439,0f000001,0*15507eb4\n\tsystem status\tnormal 2 27.900000 0 0\trobot status\t229.646824\t104.848439\t8.253000\t0.103360\t-1.313771\t169.575614\t0.357000\t-0.093000\n\t\n15:37:07.2\tlog_raw\tgps_raw\t#INSPVAXA,USB3,0,50.5,FINESTEERING,2107,283045.200,02000000,471d,15824;INS_ALIGNMENT_COMPLETE,INS_RTKFIXED,37.37107528342,126.72342611252,8.2498,22.3000,0.0937,-0.2667,-0.0213,0.106140982,-1.381356715,280.387415743,0.4469,0.2952,0.5622,0.1142,0.0926,0.0779,0.0977,0.1027,4.9453,0f000001,0*b33463af\n\tsystem status\tnormal 2 27.900000 0 0\trobot status\t229.507194\t104.886944\t8.249800\t0.106141\t-1.381357\t169.612584\t0.272000\t0.034000\n\t\n15:37:07.7\tlog_raw\tgps_raw\t#INSPVAXA,USB3,0,50.5,FINESTEERING,2107,283045.700,02000000,471d,15824;INS_ALIGNMENT_COMPLETE,INS_RTKFIXED,37.37107563193,126.72342458286,8.2474,22.3000,0.0924,-0.2735,-0.0177,0.170304952,-1.470111743,280.394073740,0.4469,0.2952,0.5622,0.1142,0.0926,0.0779,0.0977,0.1027,4.9453,0f000001,0*1961b7fd\n\tsystem status\tnormal 2 27.900000 0 0\trobot status\t229.371699\t104.925627\t8.247400\t0.170305\t-1.470112\t169.605926\t0.212000\t0.128000\n\t\n15:37:08.2\tlog_raw\tgps_raw\t#INSPVAXA,USB3,0,50.5,FINESTEERING,2107,283046.200,02000000,471d,15824;INS_ALIGNMENT_COMPLETE,INS_RTKFIXED,37.37107597691,126.72342305519,8.2441,22.3000,0.1009,-0.2727,-0.0163,0.064516230,-1.445309822,280.441255220,0.4468,0.2952,0.5622,0.1142,0.0926,0.0779,0.0977,0.1027,4.9463,0f000001,0*2fb8f12d\n\tsystem status\tnormal 2 27.900000 0 0\trobot status\t229.236380\t104.963918\t8.244100\t0.064516\t-1.445310\t169.558745\t0.395000\t-0.154000\n\t\n15:37:08.7\tlog_raw\tgps_raw\t#INSPVAXA,USB3,0,50.5,FINESTEERING,2107,283046.700,02000000,471d,15824;INS_ALIGNMENT_COMPLETE,INS_RTKFIXED,37.37107633807,126.72342148609,8.2393,22.3000,0.0964,-0.2701,-0.0237,0.142828427,-1.613985055,280.469492916,0.4468,0.2952,0.5622,0.1142,0.0926,0.0779,0.0977,0.1027,4.9463,0f000001,0*98edc3e5\n\tsystem status\tnormal 2 27.900000 0 0\trobot status\t229.097392\t105.004005\t8.239300\t0.142828\t-1.613985\t169.530507\t0.287000\t0.009000\n\t\n15:37:09.2\tlog_raw\tgps_raw\t#INSPVAXA,USB3,0,51.0,FINESTEERING,2107,283047.200,02000000,471d,15824;INS_ALIGNMENT_COMPLETE,INS_RTKFIXED,37.37107668709,126.72341995437,8.2353,22.3000,0.0927,-0.2633,-0.0258,0.010167454,-1.546701377,280.494856873,0.4468,0.2952,0.5623,0.1142,0.0927,0.0779,0.0977,0.1028,4.9471,0f000001,0*6fb0fd0d\n\tsystem status\tnormal 2 28.000000 0 0\trobot status\t228.961715\t105.042745\t8.235300\t0.010167\t-1.546701\t169.505143\t0.261000\t0.049000\n\t\n15:37:09.7\tlog_raw\tgps_raw\t#INSPVAXA,USB3,0,51.0,FINESTEERING,2107,283047.700,02000000,471d,15824;INS_ALIGNMENT_COMPLETE,INS_RTKFIXED,37.37107702961,126.72341848936,8.2340,22.3000,0.0963,-0.2679,-0.0257,0.001855502,-1.278269974,280.498870950,0.4468,0.2952,0.5623,0.1142,0.0927,0.0779,0.0977,0.1028,4.9471,0f000001,0*57b2ac91\n\tsystem status\tnormal 2 28.000000 0 0\trobot status\t228.831947\t105.080763\t8.234000\t0.001856\t-1.278270\t169.501129\t0.297000\t-0.006000\n\t\n15:37:10.2\tlog_raw\tgps_raw\t#INSPVAXA,USB3,0,51.0,FINESTEERING,2107,283048.200,02000000,471d,15824;INS_ALIGNMENT_COMPLETE,INS_RTKFIXED,37.37107738369,126.72341697976,8.2314,22.3000,0.0870,-0.2415,-0.0190,0.047758290,-1.244931408,280.498951472,0.4468,0.2952,0.5625,0.1142,0.0926,0.0779,0.0977,0.1028,4.9478,0f000001,0*d01a0722\n\tsystem status\tnormal 2 28.000000 0 0\trobot status\t228.698229\t105.120064\t8.231400\t0.047758\t-1.244931\t169.501049\t0.275000\t0.016000\n\t\n15:37:10.7\tlog_raw\tgps_raw\t#INSPVAXA,USB3,0,51.0,FINESTEERING,2107,283048.700,02000000,471d,15824;INS_ALIGNMENT_COMPLETE,INS_RTKFIXED,37.37107774021,126.72341542793,8.2273,22.3000,0.0934,-0.2612,-0.0233,0.100861345,-1.232017596,280.548708433,0.4468,0.2952,0.5625,0.1142,0.0926,0.0779,0.0977,0.1028,4.9478,0f000001,0*f829d1eb\n\tsystem status\tnormal 2 28.000000 0 0\trobot status\t228.560770\t105.159636\t8.227300\t0.100861\t-1.232018\t169.451292\t0.269000\t0.046000\n\t\n15:37:11.2\tlog_raw\tgps_raw\t#INSPVAXA,USB3,0,51.5,FINESTEERING,2107,283049.200,02000000,471d,15824;INS_ALIGNMENT_COMPLETE,INS_RTKFIXED,37.37107809495,126.72341393568,8.2249,22.3000,0.0985,-0.2703,-0.0295,0.221283092,-1.050797782,280.593013812,0.4472,0.2952,0.5628,0.1144,0.0926,0.0779,0.0977,0.1029,4.9484,0f000001,0*0fbf0092\n\tsystem status\tnormal 2 27.900000 0 0\trobot status\t228.428589\t105.199010\t8.224900\t0.221283\t-1.050798\t169.406986\t0.309000\t-0.008000\n\t\n15:37:11.7\tlog_raw\tgps_raw\t#INSPVAXA,USB3,0,51.5,FINESTEERING,2107,283049.700,02000000,471d,15824;INS_ALIGNMENT_COMPLETE,INS_RTKFIXED,37.37107844035,126.72341241620,8.2243,22.3000,0.0876,-0.2464,-0.0197,0.278290436,-1.204720693,280.644287855,0.4472,0.2952,0.5628,0.1144,0.0926,0.0779,0.0977,0.1029,4.9484,0f000001,0*062abefc\n\tsystem status\tnormal 2 28.000000 0 0\trobot status\t228.293996\t105.237348\t8.224300\t0.278290\t-1.204721\t169.355712\t0.278000\t0.017000\n\t\n15:37:12.2\tlog_raw\tgps_raw\t#DUALANTENNAHEADINGA,USB3,0,46.0,FINESTEERING,2107,283050.200,02000000,d426,15824;INSUFFICIENT_OBS,NONE,-1.000000000,0.000000000,0.000000000,0.0,0.000000000,0.000000000,\"631T\",16,2,2,2,04,00,20,00*50cdafe2\n\tsystem status\tnormal 2 28.000000 0 0\trobot status\t228.152007\t105.276247\t8.223500\t0.141169\t-1.353172\t169.292512\t0.293000\t0.014000\n\t\n15:37:12.7\tlog_raw\tgps_raw\t#INSPVAXA,USB3,0,46.0,FINESTEERING,2107,283050.700,02000000,471d,15824;INS_ALIGNMENT_COMPLETE,INS_RTKFIXED,37.37107913318,126.72340926618,8.2224,22.3000,0.0989,-0.2842,-0.0266,-0.029207356,-1.258376136,280.779017967,0.4478,0.2954,0.5630,0.1143,0.0926,0.0779,0.0977,0.1029,4.9492,0f000001,0*5132ab61\n\tsystem status\tnormal 2 28.000000 0 0\trobot status\t228.014972\t105.314249\t8.222400\t-0.029207\t-1.258376\t169.220982\t0.324000\t-0.012000\n\t\n15:37:13.2\tlog_raw\tgps_raw\t#DUALANTENNAHEADINGA,USB3,0,49.5,FINESTEERING,2107,283051.200,02000000,d426,15824;INSUFFICIENT_OBS,NONE,-1.000000000,0.000000000,0.000000000,0.0,0.000000000,0.000000000,\"631T\",13,2,2,2,04,00,20,00*248e5ed2\n\tsystem status\tnormal 2 27.900000 0 0\trobot status\t227.880257\t105.352709\t8.221700\t0.048821\t-1.285395\t169.456184\t0.260000\t0.093000\n\t\n15:37:13.7\tlog_raw\tgps_raw\t#DUALANTENNAHEADINGA,USB3,0,49.5,FINESTEERING,2107,283051.700,02000000,d426,15824;INSUFFICIENT_OBS,NONE,-1.000000000,0.000000000,0.000000000,0.0,0.000000000,0.000000000,\"631T\",14,2,2,2,04,00,20,00*b9a3c4c0\n\tsystem status\tnormal 2 27.900000 0 0\trobot status\t227.739909\t105.391302\t8.220300\t0.300573\t-1.403055\t169.900669\t0.408000\t-0.149000\n\t\n15:37:14.2\tlog_raw\tgps_raw\t#INSPVAXA,USB3,0,50.5,FINESTEERING,2107,283052.200,02000000,471d,15824;INS_ALIGNMENT_COMPLETE,INS_RTKFIXED,37.37108016490,126.72340456105,8.2187,22.3000,0.0964,-0.2582,-0.0125,0.437479141,-1.522113424,279.604758230,0.4484,0.2957,0.5640,0.1144,0.0927,0.0779,0.0976,0.1029,4.9509,0f000001,0*77064c2d\n\tsystem status\tnormal 2 27.800000 0 0\trobot status\t227.598200\t105.428765\t8.218700\t0.437479\t-1.522113\t170.395242\t0.230000\t0.131000\n\t\n15:37:14.7\tlog_raw\tgps_raw\t#INSPVAXA,USB3,0,50.5,FINESTEERING,2107,283052.700,02000000,471d,15824;INS_ALIGNMENT_COMPLETE,INS_RTKFIXED,37.37108046861,126.72340298306,8.2170,22.3000,0.0891,-0.2658,-0.0140,0.468373429,-1.552166741,279.130645467,0.4484,0.2957,0.5640,0.1144,0.0927,0.0779,0.0976,0.1029,4.9509,0f000001,0*1c6e477e\n\tsystem status\tnormal 2 27.800000 0 0\trobot status\t227.458424\t105.462476\t8.217000\t0.468373\t-1.552167\t170.869355\t0.230000\t0.127000\n\t\n15:37:15.2\tlog_raw\tgps_raw\t#INSPVAXA,USB3,0,48.5,FINESTEERING,2107,283053.200,02000000,471d,15824;INS_ALIGNMENT_COMPLETE,INS_RTKFIXED,37.37108075231,126.72340140427,8.2151,22.3000,0.0764,-0.2907,-0.0105,0.358370725,-1.600173784,278.606485761,0.4480,0.2956,0.5639,0.1143,0.0926,0.0779
